vi "Receive Data.vi"(8 "error in (no error)":errorcluster, 9 "timeout ms (25000)":i32=25000, 11 "UDP Network Connection in":refnum<k16>) -> (0 "error out":errorcluster, 1 "Chunks Dropped":bool, 3 "Data":string)   [LabVIEW 2017]
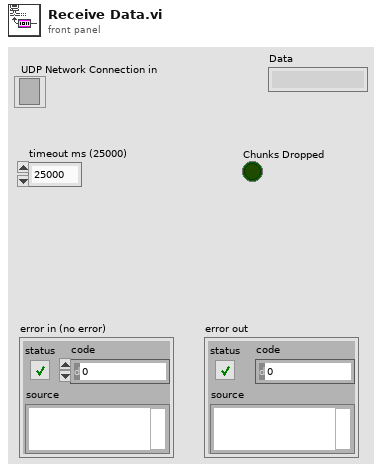
[diagram p1: front panel]
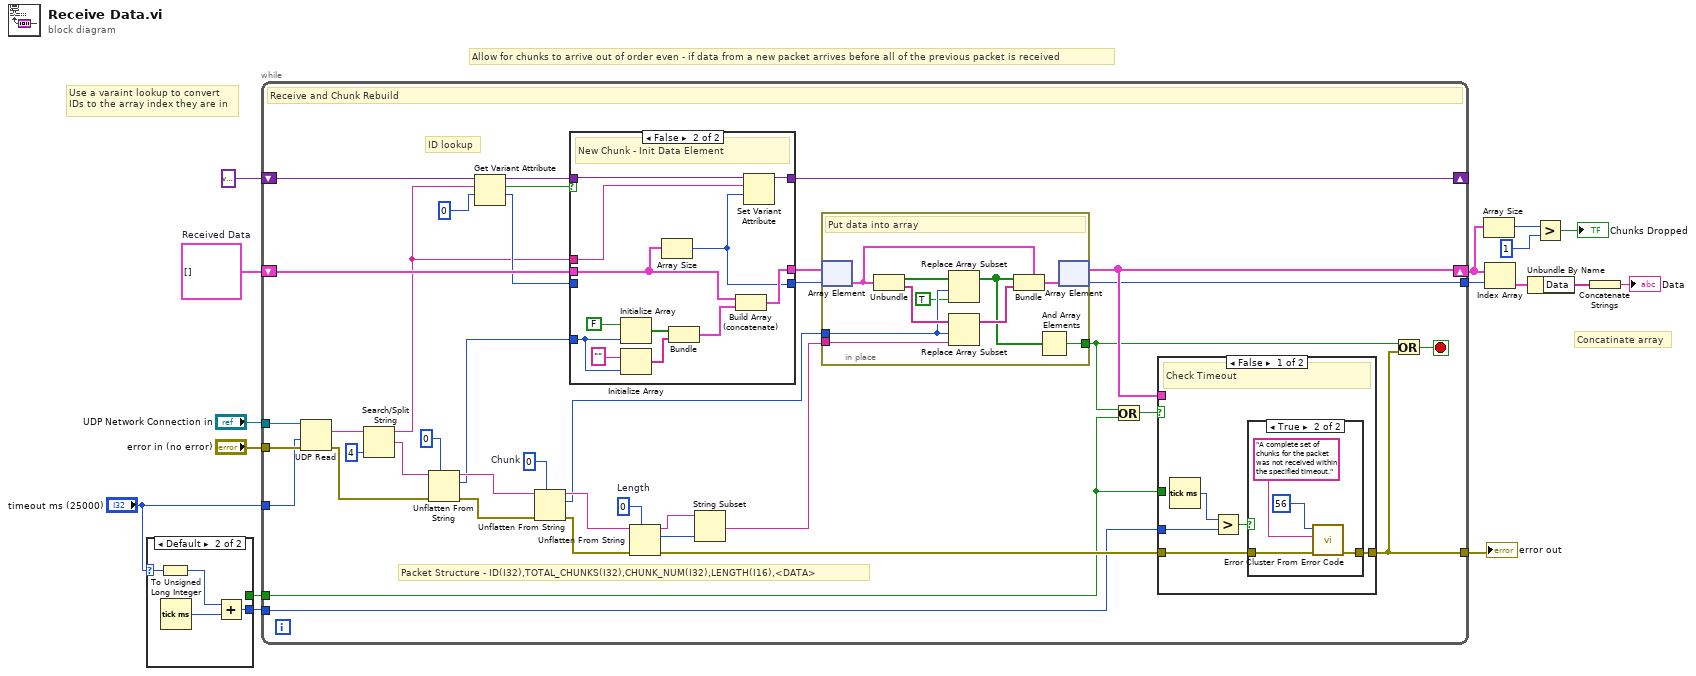
[diagram p0: block diagram]
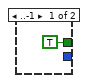
[diagram p2: hidden frame]
diagram:
  w14 = cluster{"Rec.":bool[], "Data":string[]}[] []  # Received Data
  # "Concatinate array"
  # "Use a varaint lookup to convert\nIDs to the array index they are in"
  # "Allow for chunks to arrive out of order even - if data from a new packet arrives before all of the previous packet is received"
  n1 = case shown="Default" "timeout ms (25000)" {
    selector: "timeout ms (25000)" -> [_ w19]
    tunnel: [_ w20] -> w12
    tunnel: [TRUE _] -> w10
    frame ..-1 {
    }
    frame Default {
      n2 = To Unsigned Long Integer(number=w19) -> (unsigned 32bit integer=w18:u32)
      n3 = Tick Count (ms)() -> (millisecond timer value=w21:u32)
      n4 = Add(x=w18, y=w21) -> (x+y=w20:u32)
    }
  }
  n5 = while {
    tunnel: "error in (no error)" -> [w49]
    tunnel: "UDP Network Connection in" -> [w59]
    tunnel: "timeout ms (25000)" -> [w28]
    shift-right: [w30] -> w4
    shift-left: w14 -> [w40]
    shift-right: [w37] -> _
    shift-left: variant -> [w43]
    tunnel: w12 -> [w29]
    tunnel: w10 -> [w26]
    tunnel: [w23] -> w9
    tunnel: [w22] -> w5
    stop <- w24 stop-if-true
    w52 = u16 0  # Length
    w56 = 0  # Chunk
    # "ID lookup"
    # "Packet Structure - ID(I32),TOTAL_CHUNKS(I32),CHUNK_NUM(I32),LENGTH(I16),<DATA>"
    # "Receive and Chunk Rebuild"
    n6 = UDP Read(connection ID=w59, timeout ms (25000)=w28, 8:w49) -> (data out=w47:string, error out=w44:errorcluster)  [unwired: 1 in, 3 out]
    n7 = Search/Split String(string=w47, offset (0)=4) -> (substring before match=w36:string, match + rest of string=w45:string)  [unwired: 1 in, 1 out]
    n8 = Unflatten From String(type=0, binary string=w45, error in (no error)=w44) -> (rest of the binary string=w57:string, value=w48:i32, error out=w58:errorcluster)  [unwired: 2 in]
    n9 = Get Variant Attribute(Variant=w43, name=w36, default value (empty Variant)=0) -> (duplicate Variant=w38:variant, found=w41:bool, value=w39:i32)  [unwired: 1 in, 1 out]
    n10 = Unflatten From String(type=w56, binary string=w57, error in (no error)=w58) -> (rest of the binary string=w53:string, value=w33:i32, error out=w54:errorcluster)  [unwired: 2 in]
    n11 = case shown="False" w41 {
      tunnel: w48 -> [_ w84]
      tunnel: w40 -> [w82 w85]
      tunnel: w39 -> [w83 _]
      tunnel: [w82 w91] -> w35
      tunnel: [w83 w87] -> w34
      tunnel: w38 -> [w81 w88]
      tunnel: [w81 w89] -> w37
      tunnel: w36 -> [_ w86]
      frame True {
        # "Currently Rebuilding"
      }
      frame False {
        # "New Chunk - Init Data Element"
        n12 = Initialize Array(FALSE, w84) -> (w93:bool[])
        n13 = Initialize Array("", w84) -> (w92:string[])
        n14 = Array Size(array=w85) -> (size(s)=w87:i32)
        n15 = Bundle(w93, w92) -> (w90:cluster{bool[], string[]})  [unwired: 1 in]
        n16 = Build Array (concatenate)(w85, w90) -> (w91:cluster{"Rec.":bool[], "Data":string[]}[])
        n17 = Set Variant Attribute(Variant=w88, name=w86, value=w87) -> (Variant out=w89:variant)  [unwired: 1 in, 2 out]
      }
    }
    n18 = Unflatten From String(type=w52, binary string=w53, error in (no error)=w54) -> (rest of the binary string=w51:string, value=w50:u16, error out=w31:errorcluster)  [unwired: 2 in]
    n19 = String Subset(string=w51, length (rest)=w50) -> (substring=w32:string)  [unwired: 1 in]
    n20 = in-place {
      in-place-border: w33 -> [w78]
      in-place-border: w32 -> [w74]
      in-place-border: [w72] -> w25
      # "Put data into array"
      n21 = in-place-array #1(w35, w34) -> (w75:cluster{"Rec.":bool[], "Data":string[]})
      n22 = Unbundle(w75) -> ("Rec."=w80:bool[], "Data"=w79:string[])
      n23 = Replace Array Subset(array=w80, new element=TRUE ("new element/subarray"), index=w78) -> (w73:bool[])
      n24 = Replace Array Subset(array=w79, new element=w74, index=w78) -> (w76:string[])
      n25 = Bundle(cluster=w75, "Rec."=w73, "Data"=w76) -> (w77:cluster{"Rec.":bool[], "Data":string[]})
      n26 = And Array Elements(Boolean array=w73) -> (logical AND=w72:bool)
      n27 = in-place-array #1(w77) -> (w30:cluster{"Rec.":bool[], "Data":string[]}[], w23:i32)
    }
    n28 = Or(x=w25, y=w26) -> (x .or. y?=w27:bool)
    n29 = case shown="False" w27 {
      tunnel: w31 -> [w61 w70]
      tunnel: w30 -> [_ _]
      tunnel: w29 -> [w63 _]
      tunnel: w26 -> [_ _]
      tunnel: [w60 w70] -> w22
      frame False {
        # "Check Timeout"
        n30 = Tick Count (ms)() -> (millisecond timer value=w64:u32)
        n31 = Greater?(x=w64, y=w63) -> (0:w62:bool)
        n32 = case shown="True" w62 {
          tunnel: w61 -> [w65 w69]
          tunnel: [w65 w68] -> w60
          frame False {
          }
          frame True {
            n33 = call <vilib>:"Error Cluster From Error Code.vi"("error in (no error)"=w69, "error message (\"\")"="A complete set of chunks for the packet was not received within the specified timeout." ("error message (\"\")"), "error code (0)"=56) -> ("error out"=w68:errorcluster)  [unwired: 6 in]
          }
        }
      }
      frame True {
        # "Ignore Timeout"
      }
    }
    n34 = Or(x=w25, y=w22) -> (x .or. y?=w24:bool)
  }
  "error out" <- w5
  n35 = Array Size(array=w4) -> (size(s)=w3:i32)
  n36 = Index Array(array=w4, index=w9) -> (element=w8:cluster{"Rec.":bool[], "Data":string[]})
  n37 = Unbundle By Name(w8) -> ("Data"=w7:string[])
  n38 = Greater?(x=w3, y=1) -> (0:→"Chunks Dropped":bool)
  n39 = Concatenate Strings(w7) -> (→"Data":string)
